vi "CountHigh10.vi"(10 "10bit input":bool[](array[boolean])=[FALSE, FALSE, FALSE, FALSE, FALSE, FALSE, FALSE, FALSE, FALSE, FALSE]) -> (2 "No. of detected high":u16)   [LabVIEW 2012]
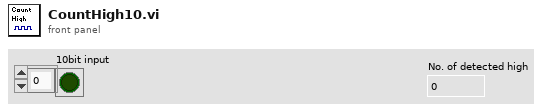
[diagram p1: front panel]
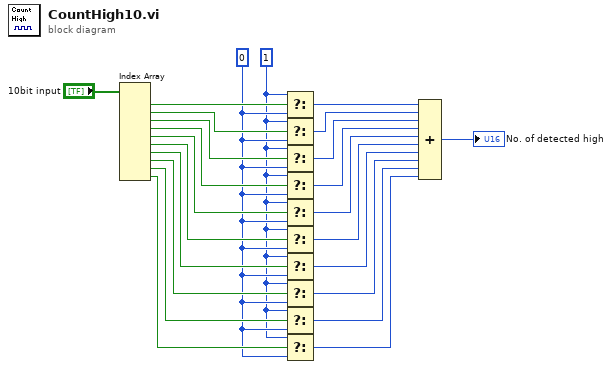
[diagram p0: block diagram]
diagram:
  w10 = u16 1
  w11 = u16 0
  n1 = Index Array(array="10bit input") -> (element #1=w22:bool, element #2=w21:bool, element #3=w20:bool, element #4=w19:bool, element #5=w18:bool, element #6=w17:bool, element #7=w16:bool, element #8=w15:bool, element #9=w14:bool, element #10=w13:bool)  [unwired: 10 in]
  n2 = Select(t=w10, s=w22, f=w11) -> (s? t:f=w12:u16)
  n3 = Select(t=w10, s=w21, f=w11) -> (s? t:f=w9:u16)
  n4 = Select(t=w10, s=w20, f=w11) -> (s? t:f=w8:u16)
  n5 = Select(t=w10, s=w19, f=w11) -> (s? t:f=w7:u16)
  n6 = Select(t=w10, s=w18, f=w11) -> (s? t:f=w6:u16)
  n7 = Select(t=w10, s=w17, f=w11) -> (s? t:f=w5:u16)
  n8 = Select(t=w10, s=w16, f=w11) -> (s? t:f=w4:u16)
  n9 = Select(t=w10, s=w15, f=w11) -> (s? t:f=w3:u16)
  n10 = Select(t=w10, s=w14, f=w11) -> (s? t:f=w2:u16)
  n11 = Select(t=w10, s=w13, f=w11) -> (s? t:f=w1:u16)
  n12 = Compound Arithmetic op=ADD(w12, w9, w8, w7, w6, w5, w4, w3, w2, w1) -> (→"No. of detected high":u16)
